vi "Hybrid Test Stand Instrumentation.vi"() -> ()   [LabVIEW 2020]
uses:
  <vilib>/Utility/TDMS File Viewer/NI_TDMS File Viewer.lvlib
panel:
  out "Stream Parameters":T1 {"Device Backlog [%]" format="%.2f"}
  out "Actual Scan Rate (Hz)":dbl=1000.0 format="%.3f"
  in  "AIN Range":u8(ring) items=["LJ_rgBIP10V", "LJ_rgBIP1V", "LJ_rgBIPP1V", "LJ_rgBIPP01V"]
  in  "Display Rate (Hz)":i32=1
  in  "Binary":bool
  in  "StreamSettlingFactor":i32
  in  "Resolution Index":u8
  in  "PC buffer size (seconds)":dbl=10.0 format="%.2f"
  in  "Scan Rate (Hz)":dbl=1000.0 format="%.3f"
  out "Oxidizer Mass Flow":dbl(graph)
  out "N2O Tank Mass":dbl(slide) scale=17.0..21.0
  out "Grain Center":dbl(slide) scale=-70.0..40.0
  out "Post-Combustion":dbl(slide) scale=-70.0..40.0
  out "Pre-Combustion":dbl(slide) scale=-70.0..40.0
  out "Tank":dbl(slide) scale=-70.0..40.0
  out "Pressure Chart":dynamicdata(graph)
  out "Thrust Chart":dbl(graph)
  out "Run Tank Pressure":dbl(knob) scale=0.0..10.0
  out "N Flow Pressure":dbl(knob) scale=0.0..10.0
  out "N2O Flow Pressure":dbl(knob) scale=0.0..10.0
  in  "Injector":string
  in  "Orifice Size":string
  in  "File Name":string
  out "Boolean":bool
  in  "START":bool
  in  "[ESC]":bool
  out "Error Message":string
  out "error out":errorcluster
  in  "Folder Path":path
  # "UVR Instrumentation Testing"
  # "Acquires multiple analog input channels over USB from the first found U6."
  # "LJ_rgBIP10V\nLJ_rgBIP1V\nLJ_rgBIPP1V\nLJ_rgBIPP01V"
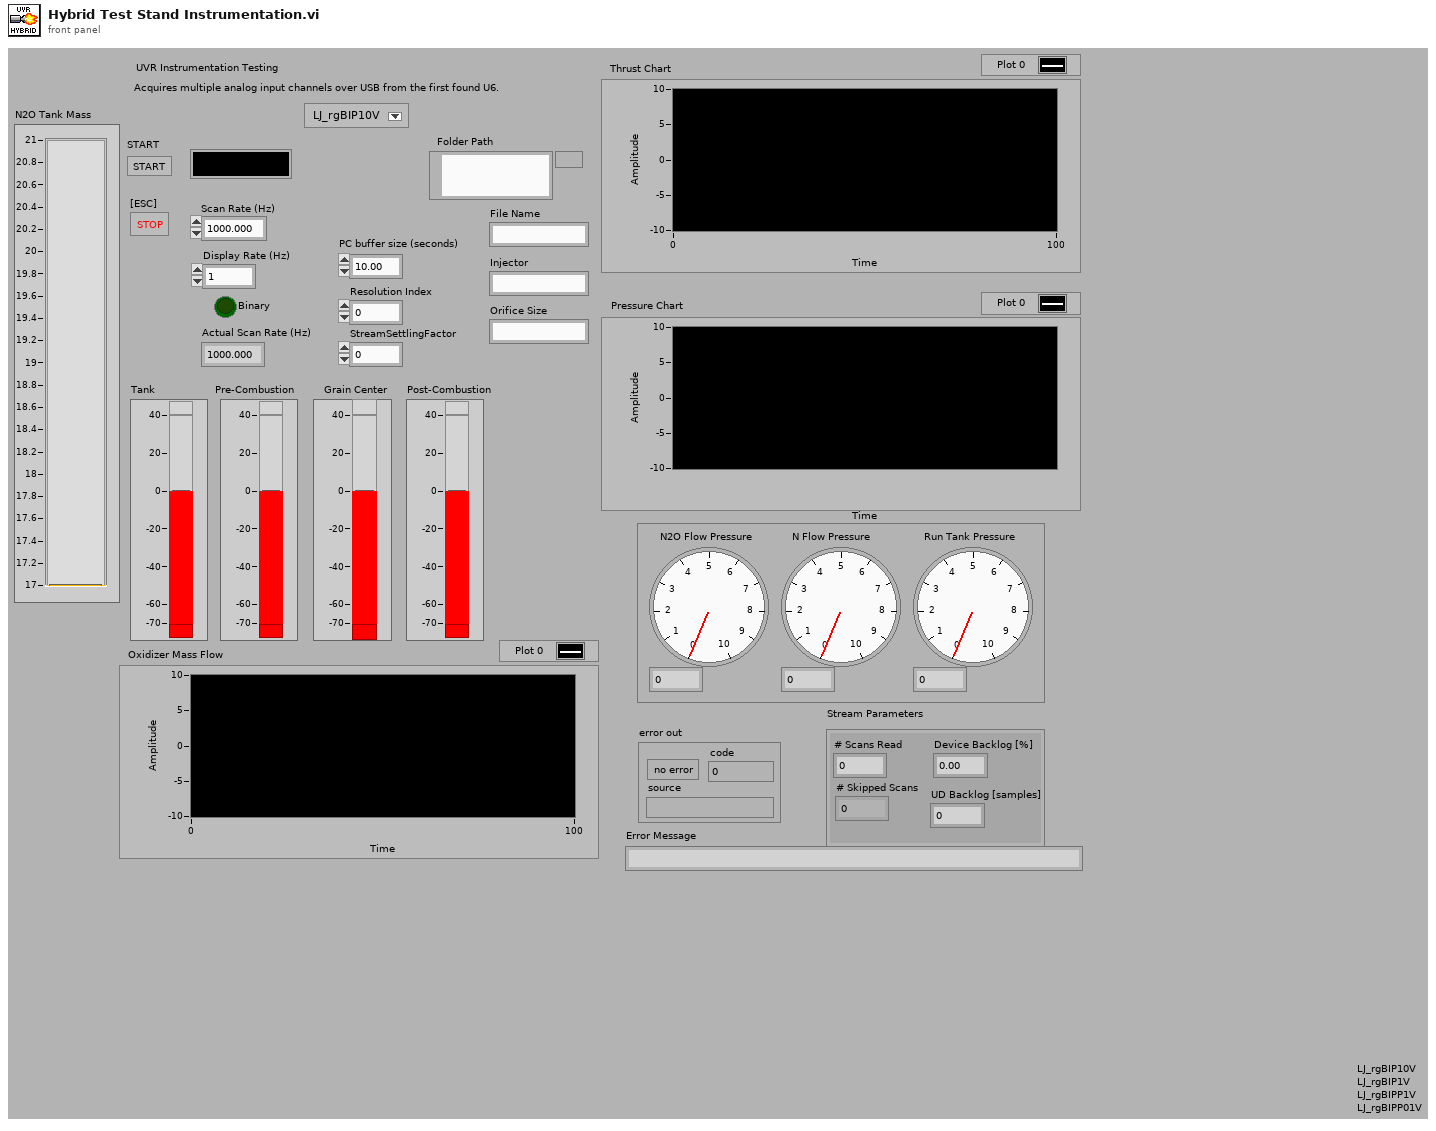
[diagram p1: front panel]
types:
  T1 = cluster{"# Scans Read":i32, "# Skipped Scans":i32, "Device Backlog [%]":dbl, "UD Backlog [samples]":i32}
  T2 = enum16{"open", "open or create", "create or replace", "create", "open (read-only)"}
  T3 = cluster{"PC buffer size (seconds)":dbl, "Resolution Index":u8, "StreamSettlingFactor":i32, "Binary":bool}
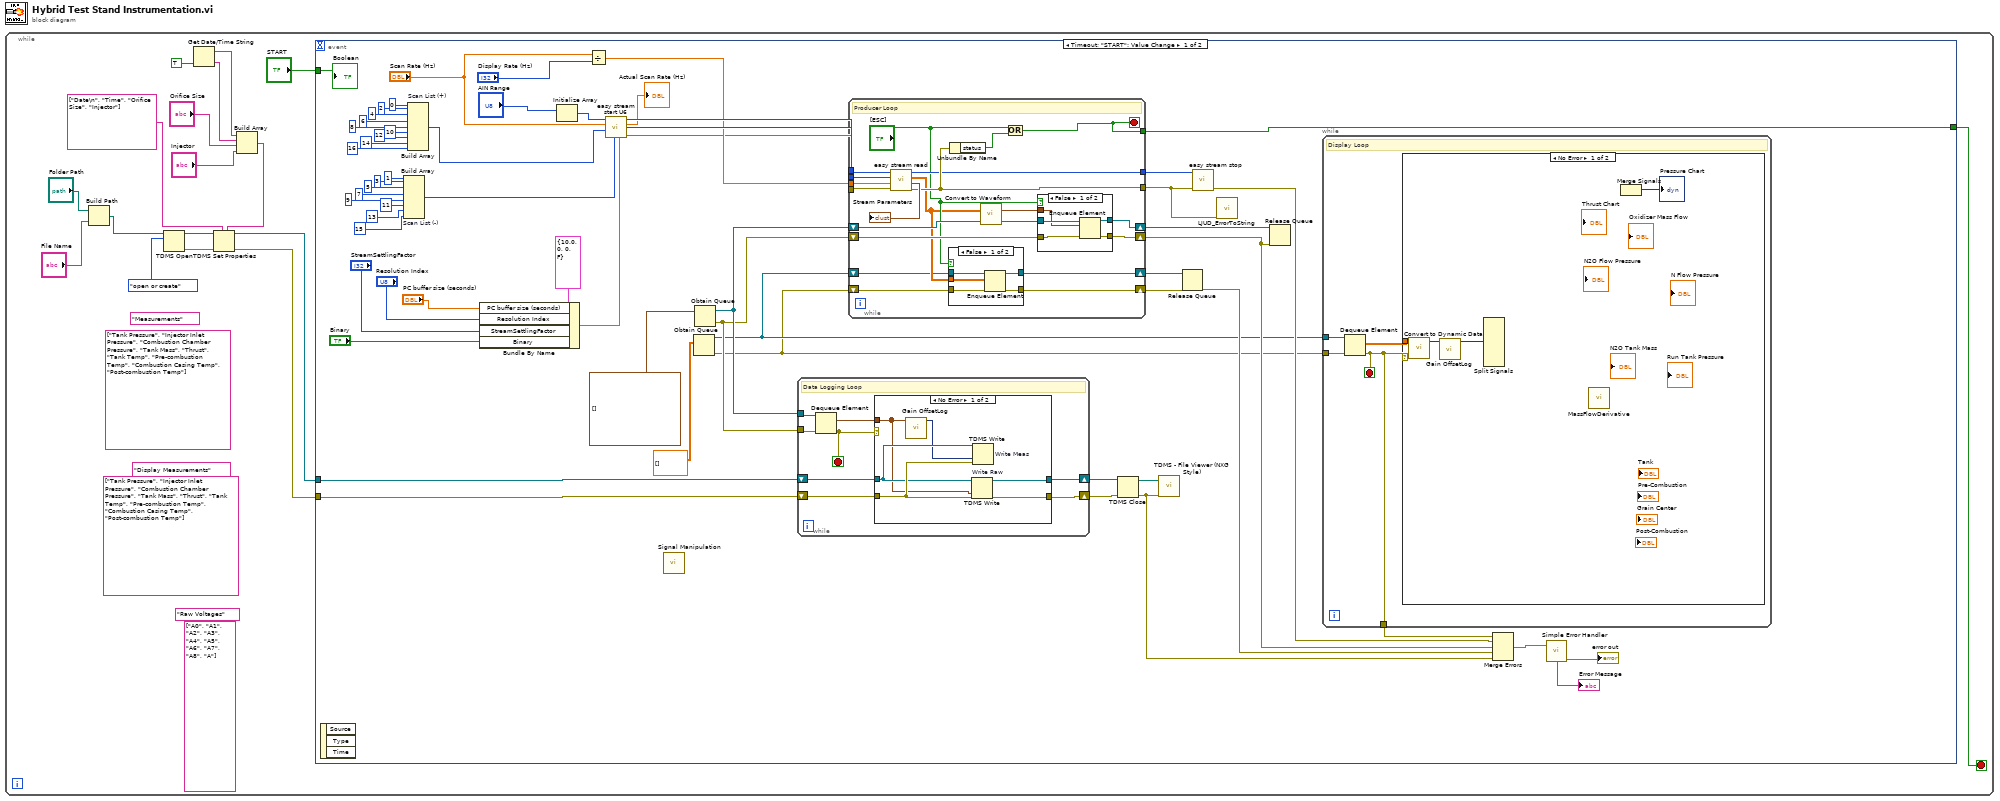
[diagram p0: block diagram]
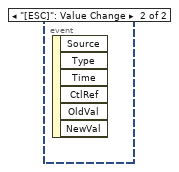
[diagram p6: hidden frame]
diagram:
  n1 = while {
    stop <- w7 stop-if-true
    (unwired) string[] ["Tank Pressure", "Injector Inlet Pressure", "Combustion Chamber Pressure", "Tank Mass", "Thrust", "Tank Temp", "Pre-combustion Temp", "Combustion Casing Temp", "Post-combustion Temp"] ("property names")
    (unwired) "Display Measurements"
    (unwired) string[] ["Tank Pressure", "Injector Inlet Pressure", "Combustion Chamber Pressure", "Tank Mass", "Thrust", "Tank Temp", "Pre-combustion Temp", "Combustion Casing Temp", "Post-combustion Temp"] ("property names")
    (unwired) "Measurements"
    (unwired) string[] ["A0", "A1", "A2", "A3", "A4", "A5", "A6", "A7", "A8", "A"] ("property names")
    (unwired) "Raw Voltages"
    n2 = Build Path(base path="Folder Path", name or relative path="File Name") -> (appended path=w5:path)
    n3 = TDMS Open(10:T2."open or create" ("operation (0:open)"), 11:w5) -> (0:w17:errorcluster, 3:w16:refnum<k34>)  [unwired: 5 in]
    n4 = Get Date/Time String(want seconds? (F)=TRUE) -> (date string=w14:string, time string=w3:string)  [unwired: 2 in]
    n5 = Build Array(w14, w3, "Orifice Size", "Injector") -> (w12:string[])
    n6 = TDMS Set Properties(5:w12, 7:string[] ["Date\n", "Time", "Orifice Size", "Injector"] ("property names"), 8:w17, 11:w16) -> (0:w9:errorcluster, 3:w10:refnum<k34>)  [unwired: 2 in, 2 out]
    n7 = event shown="[0] Timeout;  \"START\": Value Change" {
      selector: _ -> [_ _]
      dyn-events: _ -> [_ _]
      timeout: _ -> [_ _]
      tunnel: w10 -> [w65 _]
      tunnel: w9 -> [w76 _]
      tunnel: "START" -> [w77 _]
      tunnel: [w74 _] -> w7
      event Timeout; "START": Value Change {
        n8 = event-data() -> ()  [unwired: 1 in, 3 out]
        n9 = Build Array "Scan List (-)"(1 ("SettlingFactor"), 3 ("SettlingFactor"), 5 ("SettlingFactor"), 7 ("SettlingFactor"), 9 ("SettlingFactor"), 11 ("SettlingFactor"), 13 ("SettlingFactor"), 15 ("SettlingFactor")) -> (w37:i32[])
        n10 = Build Array "Scan List (+)"(0 ("SettlingFactor"), 2 ("SettlingFactor"), 4 ("SettlingFactor"), 6 ("SettlingFactor"), 8 ("SettlingFactor"), 10 ("SettlingFactor"), 12 ("SettlingFactor"), 14 ("SettlingFactor"), 16 ("SettlingFactor")) -> (w46:i32[])
        n11 = Bundle By Name(cluster=T3 {"PC buffer size (seconds)"=10.0, "Resolution Index"=0, "StreamSettlingFactor"=0, "Binary"=FALSE} ("Advanced"), "PC buffer size (seconds)"="PC buffer size (seconds)", "Resolution Index"="Resolution Index", "StreamSettlingFactor"="StreamSettlingFactor", "Binary"="Binary") -> (w59:T3)
        n12 = Initialize Array("AIN Range") -> (w49:u8[])  [unwired: 1 in]
        n13 = Divide(x="Scan Rate (Hz)", y="Display Rate (Hz)") -> (x/y=w31:dbl)
        n14 = call "easy stream start U6.vi"("Advanced"=w59, "Scan List (-)"=w37, "Scan List (+)"=w46, "Scan Rate (Hz)"="Scan Rate (Hz)", "Range Constants"=w49) -> ("error out"=w30:errorcluster, "# Channels"=w32:i32, "Actual Scan Rate (Hz)"=→"Actual Scan Rate (Hz)":dbl, "Handle Out"=w34:i32)  [unwired: 3 in]
        n15 = call "Signal Manipulation.vi"() -> ()  [unwired: 11 in, 1 out]
        n16 = Obtain Queue(element data type=dbl[][] []) -> (queue out=w19:refnum<queue>, error out=w18:errorcluster)  [unwired: 4 in, 1 out]
        n17 = Obtain Queue(element data type=waveform(dbl)[] [] ("Waveform")) -> (queue out=w69:refnum<queue>, error out=w68:errorcluster)  [unwired: 4 in, 1 out]
        n18 = while {
          tunnel: w69 -> [w118]
          tunnel: w68 -> [w117]
          shift-right: [w116] -> w67
          shift-left: w65 -> [w113]
          shift-right: [w115] -> w66
          shift-left: w76 -> [w119]
          stop <- w114 stop-if-true
          # "Data Logging Loop"
          n19 = Dequeue Element(queue=w118, error in (no error)=w117) -> (element=w112:waveform(dbl)[], error out=w114:errorcluster)  [unwired: 1 in, 2 out]
          n20 = case shown="No Error" w114 {
            tunnel: w113 -> [w122 w127]
            tunnel: w119 -> [w124 w126]
            tunnel: [w125 w127] -> w116
            tunnel: [w123 w126] -> w115
            tunnel: w112 -> [w121 _]
            frame No Error {
              n21 = call "Gain OffsetLog.vi"("Dynamic Data"=w121) -> ("Dynamic Data"=w120:dynamicdata)  [unwired: 10 in]
              n22 = TDMS Write "Write Raw"(0:w122, 9:w121, 11:w124) -> (4:w125:refnum<k34>, 15:w123:errorcluster)  [unwired: 3 in, 2 out]
              n23 = TDMS Write "Write Meas"(0:w122, 9:w120, 11:w124) -> ()  [unwired: 3 in, 4 out]
            }
            frame Error {
            }
          }
        }
        n24 = while {
          tunnel: [w97] -> w74
          shift-right: [w96] -> w72
          shift-left: w69 -> [w93]
          shift-right: [w95] -> w71
          shift-left: w68 -> [w94]
          tunnel: w34 -> [w92]
          tunnel: w32 -> [w91]
          tunnel: w31 -> [w90]
          tunnel: w30 -> [w89]
          tunnel: [w86] -> w25
          tunnel: [w84] -> w28
          shift-right: [w78] -> w20
          shift-left: w19 -> [w81]
          shift-right: [w79] -> w21
          shift-left: w18 -> [w80]
          stop <- w97 stop-if-true
          # "Producer Loop"
          n25 = call "easy stream read.vi"("error in"=w89, "Scans To Read"=w90, "# Channels In Stream"=w91, "Handle In"=w92) -> ("error out"=w86:errorcluster, "Stream Parameters"=→"Stream Parameters":T1, "Data"=w82:dbl[][], "Handle Out"=w84:i32)  [unwired: 4 in]
          n26 = case shown="False" "[ESC]" {
            tunnel: w82 -> [w102 _]
            tunnel: w81 -> [w101 w104]
            tunnel: w80 -> [w100 w103]
            tunnel: [w99 w103] -> w79
            tunnel: [w98 w104] -> w78
            frame False {
              n27 = Enqueue Element(queue=w101, element=w102, error in (no error)=w100) -> (queue out=w98:refnum<queue>, error out=w99:errorcluster)  [unwired: 1 in, 1 out]
            }
            frame True {
            }
          }
          n28 = Unbundle By Name(w86) -> ("status"=w85:bool)
          n29 = call "Convert to Waveform.vi"("Data"=w82) -> ("Waveform"=w87:waveform(dbl)[])  [unwired: 10 in]
          n30 = Or(x="[ESC]", y=w85) -> (x .or. y?=w97:bool)
          n31 = case shown="False" "[ESC]" {
            tunnel: w93 -> [w109 w111]
            tunnel: [w108 w111] -> w96
            tunnel: [w107 w110] -> w95
            tunnel: w94 -> [w106 w110]
            tunnel: w87 -> [w105 _]
            frame False {
              n32 = Enqueue Element(queue=w109, element=w105, error in (no error)=w106) -> (queue out=w108:refnum<queue>, error out=w107:errorcluster)  [unwired: 1 in, 1 out]
            }
            frame True {
            }
          }
        }
        n33 = TDMS Close(8:w66, 11:w67) -> (0:w23:errorcluster, 3:w26:path)
        n34 = call <vilib>:"TDMS - File Viewer (NXG Style).vi"("error in"=w23, "file in"=w26) -> ()  [unwired: 8 in, 2 out]
        n35 = Release Queue(queue=w20, error in (no error)=w21) -> (error out=w22:errorcluster)  [unwired: 1 in, 2 out]
        n36 = call "easy stream stop.vi"("error in"=w25, "Handle In"=w28) -> ("error out"=w27:errorcluster)  [unwired: 7 in, 2 out]
        n37 = call "LJUD_ErrorToString.vi"("error in"=w25) -> ()  [unwired: 10 in, 1 out]
        n38 = Release Queue(queue=w72, error in (no error)=w71) -> ()  [unwired: 1 in, 3 out]
        n39 = while "Display Loop" {
          tunnel: [w130] -> w70
          tunnel: w19 -> [w129]
          tunnel: w18 -> [w128]
          stop <- w130 stop-if-true
          # "Display Loop"
          n40 = Dequeue Element(queue=w129, error in (no error)=w128) -> (element=w131:dbl[][], error out=w130:errorcluster)  [unwired: 1 in, 2 out]
          n41 = case shown="No Error" w130 {
            tunnel: w131 -> [w134 _]
            frame No Error {
              n42 = call "Convert to Dynamic Data"("2D Array"=w134) -> ("Dynamic Data Type"=w132:dynamicdata)  [unwired: 3 in]
              n43 = call "Gain OffsetLog.vi"("Dynamic Data"=w132) -> ("Dynamic Data"=w133:dynamicdata)  [unwired: 10 in]
              n44 = Split Signals(w133) -> ()  [unwired: 9 in, 9 out]
              n45 = call "MassFlowDerivative.vi"() -> ()  [unwired: 11 in, 1 out]
              n46 = Merge Signals() -> (→"Pressure Chart":dynamicdata)  [unwired: 2 in]
            }
            frame Error {
            }
          }
        }
        n47 = Merge Errors(w70, w27, w71, w22, w23) -> (w75:errorcluster)
        n48 = call <vilib>:"Simple Error Handler.vi"("error in (no error)"=w75) -> ("error out"=→"error out":errorcluster, "message"=→"Error Message":string)  [unwired: 4 in, 3 out]
        "Boolean" <- w77
      }
      event "[ESC]": Value Change {
        n49 = event-data() -> ()  [unwired: 1 in, 6 out]
      }
    }
  }
